vi "Resize Table 2D.vi"(11 "2D Table":refnum<vi>) -> ()   [LabVIEW 2016]
uses:
  <vilib>/addons/Software Calibration Management/XControls/TBL2D.xctl
panel:
  in  "Y Size":i32=2 min=2
  in  "X Size":i32=2 min=2
  in  "Cancel Button":bool
  in  "OK Button":bool
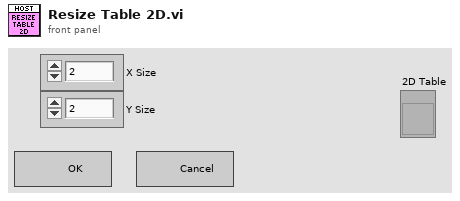
[diagram p1: front panel]
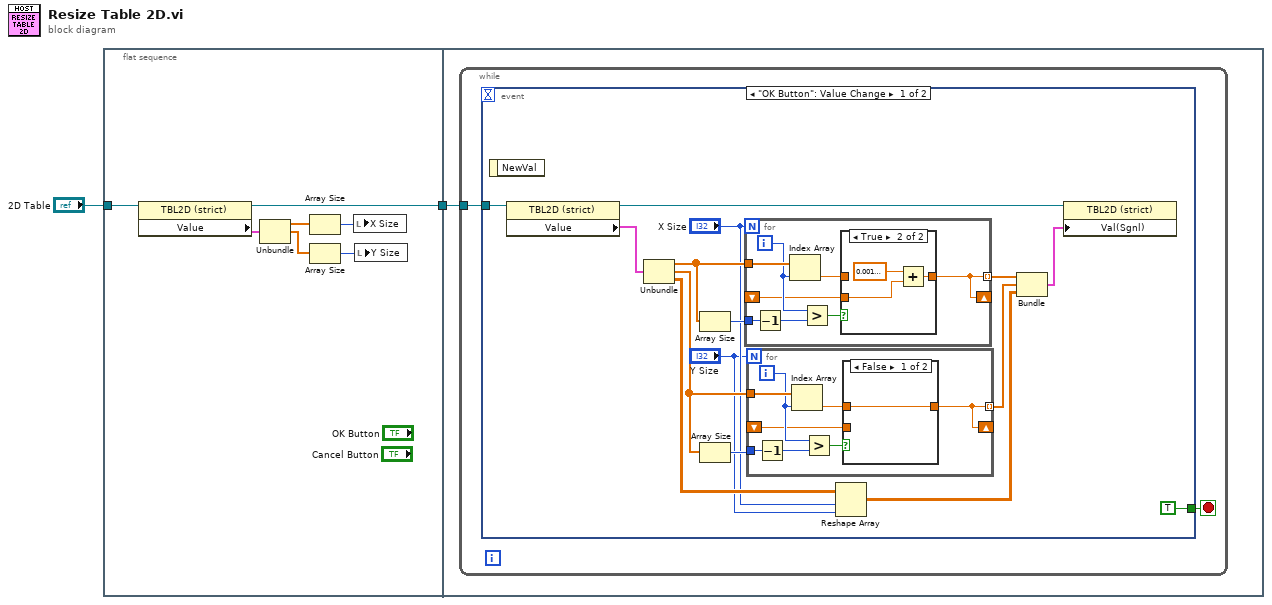
[diagram p0: block diagram]
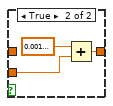
[diagram p2: hidden frame]
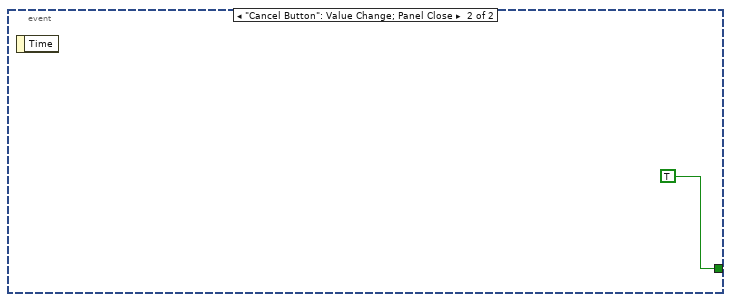
[diagram p4: hidden frame]
diagram:
  n1 = flat-sequence {
    tunnel: "2D Table" -> [w5]
    tunnel: [w3] -> w2
    tunnel: w2 -> [w10]
    frame #0 {
      n2 = property class="TBL2D (strict)"(reference=w5) -> (reference out=w3:refnum<vi>, "Value"=w4:cluster{"X":sgl[], "Y":sgl[], "Z":sgl[][]})  [unwired: 1 in, 1 out]
      n3 = Unbundle(w4) -> ("X"=w8:sgl[], "Y"=w7:sgl[])  [unwired: 1 out]
      n4 = Array Size(array=w8) -> (size(s)=w9:i32)
      n5 = Array Size(array=w7) -> (size(s)=w6:i32)
      n6 = local write "X Size"(w9) -> ()
      n7 = local write "Y Size"(w6) -> ()
    }
    frame #1 {
      n8 = while {
        tunnel: w10 -> [w11]
        stop <- w12 stop-if-true
        n9 = event shown="[0] \"OK Button\": Value Change" {
          selector: _ -> [_ _]
          dyn-events: _ -> [_ _]
          timeout: _ -> [_ _]
          tunnel: [TRUE TRUE] -> w12
          tunnel: w11 -> [w26 _]
          event "OK Button": Value Change {
            n10 = event-data() -> ()  [unwired: 1 in, 1 out]
            n11 = property class="TBL2D (strict)"(reference=w26) -> (reference out=w25:refnum<vi>, "Value"=w22:cluster{"X":sgl[], "Y":sgl[], "Z":sgl[][]})  [unwired: 1 in, 1 out]
            n12 = Unbundle(w22) -> ("X"=w23:sgl[], "Y"=w18:sgl[], "Z"=w17:sgl[][])
            n13 = Array Size(array=w23) -> (size(s)=w21:i32)
            n14 = Array Size(array=w18) -> (size(s)=w19:i32)
            n15 = for {
              N: "X Size" -> [_]
              tunnel: w23 -> [w47]
              tunnel: w21 -> [w43]
              tunnel: [w41] -> w24 mode=indexing
              shift-right: [w41] -> _
              shift-left: _ -> [w40]
              i -> [w46]
              n16 = Decrement(x=w43) -> (x-1=w42:i32)
              n17 = Index Array(array=w47, index=w46) -> (element=w44:sgl)
              n18 = Greater?(x=w46, y=w42) -> (0:w45:bool)
              n19 = case shown="True" w45 {
                tunnel: [w48 w50] -> w41
                tunnel: w44 -> [w48 _]
                tunnel: w40 -> [_ w51]
                frame False {
                }
                frame True {
                  n20 = Add(x=sgl 0.001, y=w51) -> (x+y=w50:sgl)
                }
              }
            }
            n21 = for {
              N: "Y Size" -> [_]
              tunnel: w18 -> [w35]
              tunnel: w19 -> [w31]
              tunnel: [w29] -> w20 mode=indexing
              shift-right: [w29] -> _
              shift-left: _ -> [w28]
              i -> [w34]
              n22 = Decrement(x=w31) -> (x-1=w30:i32)
              n23 = Index Array(array=w35, index=w34) -> (element=w32:sgl)
              n24 = Greater?(x=w34, y=w30) -> (0:w33:bool)
              n25 = case shown="False" w33 {
                tunnel: [w36 w38] -> w29
                tunnel: w32 -> [w36 _]
                tunnel: w28 -> [_ w39]
                frame False {
                }
                frame True {
                  n26 = Add(x=sgl 0.001, y=w39) -> (x+y=w38:sgl)
                }
              }
            }
            n27 = Reshape Array(w17, "X Size", "Y Size") -> (w16:sgl[][])
            n28 = Bundle(w24, w20, "Z"=w16) -> (w15:cluster{sgl[], sgl[], "Z":sgl[][]})  [unwired: 1 in]
            n29 = property class="TBL2D (strict)"(reference=w25, "Val(Sgnl)"=w15) -> ()  [unwired: 1 in, 2 out]
          }
          event "Cancel Button": Value Change; Panel Close {
            n30 = event-data() -> ()  [unwired: 1 in, 1 out]
          }
        }
      }
    }
  }
